vi "Socket.UDP Multicast Client.vi"() -> ()   [LabVIEW 2014]
uses:
  Classes/Socket.UDP/Socket.UDP.lvclass
  Classes/Socket.UDP/Socket.UDP.lvclass/Socket.UDP.ctl
  Classes/Socket.UDP/Accessors/Write transfer_mode.vi
panel:
  out "error out":errorcluster
  in  "Stop Button":bool
  out "Received Strings":string
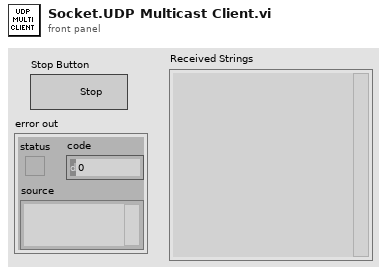
[diagram p1: front panel]
types:
  T1 = enum16{"point-to-point", "multicast", "broadcast"}
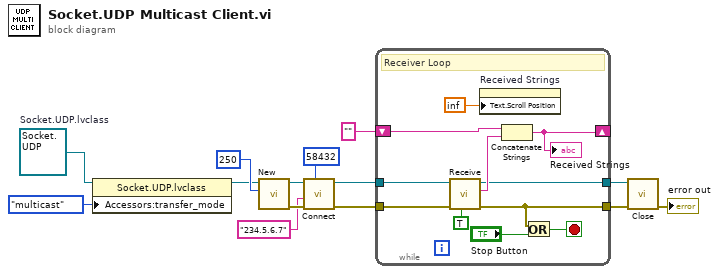
[diagram p0: block diagram]
diagram:
  w14 = refnum<class "Socket.UDP.lvclass"> refnum  # Socket.UDP.lvclass
  n1 = property class="Socket.UDP.lvclass"(reference=w14, "Accessors:transfer_mode"=T1."multicast" ("transfer_mode")) -> (reference out=w2:refnum<class "Socket.UDP.lvclass">)  [unwired: 1 in, 1 out]
  n2 = call-dynamic "New.vi"("timeout"=250, "Socket.UDP in"=w2) -> ("error out"=w12:errorcluster, "Socket.UDP out"=w11:refnum<class "Socket.UDP.lvclass">)  [unwired: 8 in]
  n3 = call-dynamic "Connect.vi"("host_port"=u16 58432, "error in (no error)"=w12, "remote_address"="234.5.6.7" ("host address"), "Socket.UDP in"=w11) -> ("error out"=w9:errorcluster, "Socket.UDP out"=w10:refnum<class "Socket.UDP.lvclass">)  [unwired: 6 in]
  n4 = while {
    tunnel: w10 -> [w21]
    tunnel: w9 -> [w22]
    shift-right: [w24] -> _
    shift-left: "" -> [w25]
    tunnel: [w18] -> w7
    tunnel: [w19] -> w6
    stop <- w17 stop-if-true
    # "Receiver Loop"
    n5 = call-dynamic "Receive.vi"("clear_timeout_error (f)"=TRUE, "error in (no error)"=w22, "Socket.UDP in"=w21) -> ("error out"=w18:errorcluster, "data out"=w20:string, "Socket.UDP out"=w19:refnum<class "Socket.UDP.lvclass">)  [unwired: 5 in, 1 out]
    n6 = property on="Received Strings" class="Str"("Text.Scroll Position"=inf) -> ()  [unwired: 2 in, 2 out]
    n7 = Concatenate Strings(w25, w20) -> (w24:string)
    "Received Strings" <- w24
    n8 = Or(x=w18, y="Stop Button") -> (x .or. y?=w17:bool)
  }
  n9 = call-dynamic "Close.vi"("error in (no error)"=w7, "Socket.UDP in"=w6) -> ("error out"=→"error out":errorcluster)  [unwired: 8 in, 1 out]
